vi "Init Data Object.vi"(11 "CRDS Data in":refnum<class "CRDS Data.lvclass">) -> (3 "CRDS Data out":refnum<class "CRDS Data.lvclass">)   [LabVIEW 2014, in "CRDS Lib.lvlib" / "CRDS Data.lvclass"]
uses:
  CRDS Data.lvclass
  Data/Data.lvlibp/Data.lvclass
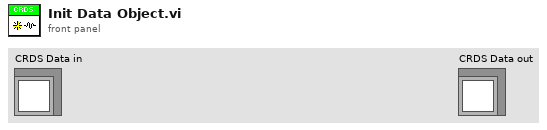
[diagram p1: front panel]
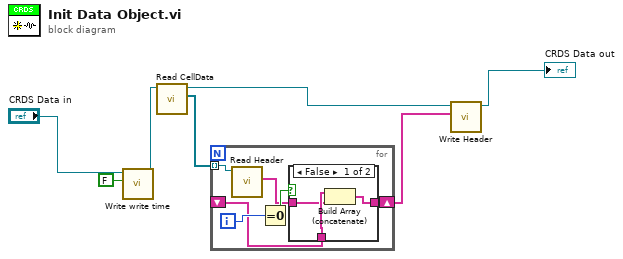
[diagram p0: block diagram]
diagram:
  n1 = call "Write write time.vi"("write time"=FALSE, "Data in"="CRDS Data in") -> ("Data out"=w5:refnum<class "CRDS Data.lvclass">)  [unwired: 8 in, 1 out]
  n2 = call "Read CellData.vi"("CRDS Data in"=w5) -> ("CellData"=w4:refnum<class "CRDS Cell Data.lvclass">[], "CRDS Data out"=w3:refnum<class "CRDS Data.lvclass">)  [unwired: 8 in, 1 out]
  n3 = for {
    tunnel: w4 -> [w13] mode=indexing
    shift-right: [w9] -> w2
    shift-left: _ -> [w8]
    i -> [w12]
    n4 = call "Read Header.vi"("Data in"=w13) -> ("Header"=w10:string[])  [unwired: 8 in, 2 out]
    n5 = Equal To 0?(x=w12) -> (x = 0?=w11:bool)
    n6 = case shown="False" w11 {
      tunnel: w10 -> [w15 w17]
      tunnel: [w14 w17] -> w9
      tunnel: w8 -> [w16 _]
      frame False {
        n7 = Build Array (concatenate)(w16, w15) -> (w14:string[])
      }
      frame True {
      }
    }
  }
  n8 = call "Write Header.vi"("Header"=w2, "Data in"=w3) -> ("Data out"=→"CRDS Data out":refnum<class "CRDS Data.lvclass">)  [unwired: 8 in, 1 out]
